vi "EoL String.vi"() -> (2 "EoL String Length":i32, 3 "EoL String":string)   [LabVIEW 2019, in "JKI JSON Serialization.lvlib" / "JSON Serializer.lvclass"]
doc: "JKI JSON 1.1.10.37\nTomi Maila - JKI\nCopyright (c) 2017, JKI"
uses:
  JSON Serializer.lvclass
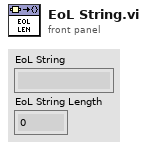
[diagram p1: front panel]
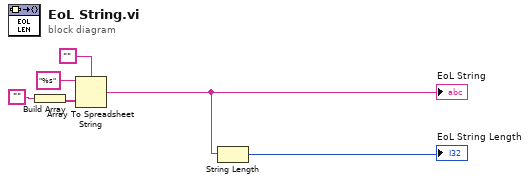
[diagram p0: block diagram]
diagram:
  n1 = Build Array("") -> (w6:string[])
  n2 = Array To Spreadsheet String(delimiter (Tab)="", array=w6, 3:"%s" ("format string")) -> (spreadsheet string=w2:string)
  "EoL String" <- w2
  n3 = String Length(string=w2) -> (length=→"EoL String Length":i32)
